vi "Create Replacement Endpoint.vi"(8 "position":T1, 9 "tunnel term":refnum<vi>) -> (3 "endpt":refnum<vi>)   [LabVIEW 2020, in "NI_TargetHelper.lvlib"]
uses:
  <vilib>/TargetSupport/NI_TargetHelper/NI_TargetHelper.lvlib
  <vilib>/Utility/miscctls.llb/LVPositionTypeDef.ctl
  <resource>/ChannelSupport/_ChannelScriptingSupport/_ChannelScriptingSupport.lvlib
  <vilib>/Utility/Data Type/NI_Data Type.lvlib
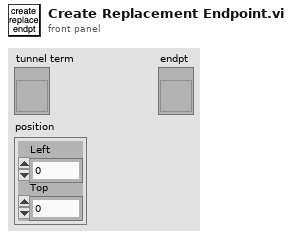
[diagram p1: front panel]
types:
  T1 = typedef "LVPositionTypeDef.ctl" = cluster{"Left":i32, "Top":i32}
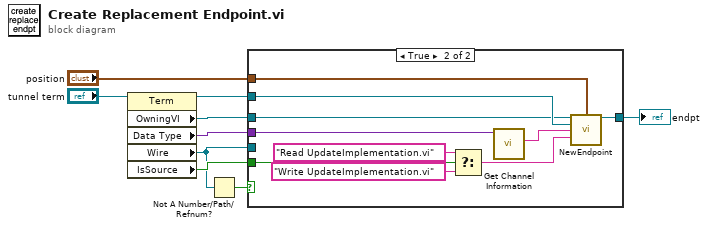
[diagram p0: block diagram]
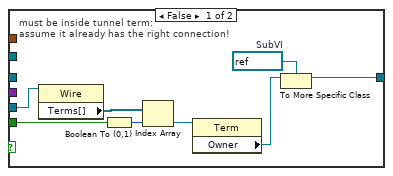
[diagram p2: hidden frame]
diagram:
  n1 = property class="Term"(reference="tunnel term") -> (reference out=w6:refnum<vi>, "OwningVI"=w3:refnum<vi>, "Data Type"=w8:variant, "Wire"=w2:refnum<vi>, "IsSource"=w9:bool)  [unwired: 1 in, 1 out]
  n2 = Not A Number/Path/Refnum?(number/path/refnum=w2) -> (NaN/Path/Refnum?=w7:bool)
  n3 = case shown="True" w7 {
    tunnel: w6 -> [_ w27]
    tunnel: "position" -> [_ w20]
    tunnel: w9 -> [w15 w23]
    tunnel: w8 -> [_ w22]
    tunnel: w3 -> [_ w19]
    tunnel: w2 -> [w17 _]
    tunnel: [w11 w18] -> w1
    frame False {
      w10 = refnum<vi> refnum  # SubVI
      # "must be inside tunnel term:\nassume it already has the right connection!"
      n4 = property class="Wire"(reference=w17) -> ("Terms[]"=w16:refnum<vi>[])  [unwired: 1 in, 2 out]
      n5 = Boolean To (0,1)(Boolean=w15) -> (0, 1=w14:i16)
      n6 = Index Array(array=w16, index=w14) -> (element=w13:refnum<vi>)
      n7 = property class="Term"(reference=w13) -> ("Owner"=w12:refnum<vi>)  [unwired: 1 in, 2 out]
      n8 = To More Specific Class(target class=w10, reference=w12) -> (specific class reference=w11:refnum<vi>)  [unwired: 1 in, 1 out]
    }
    frame True {
      n9 = Select(t="Read UpdateImplementation.vi", s=w23, f="Write UpdateImplementation.vi") -> (s? t:f=w24:string)
      n10 = call <vilib>:"Get Channel Information.vi"("variant"=w22) -> ("template name"=w21:string)  [unwired: 6 in, 4 out]
      n11 = call <resource>:"NewEndpoint.vi"("VI in"=w19, "Mouse Position"=w20, "term"=w27, "Channel"=w21, "Endpoint (w Ext)"=w24) -> ("Existing or Replacement Endpoint"=w18:refnum<vi>)  [unwired: 9 in, 1 out]
    }
  }
  "endpt" <- w1
